vi "UltimateSerialMonitor.vi"() -> ()   [LabVIEW 2012]
uses:
  TypeDefs/StateCtrl.ctl
panel:
  in  "stop":bool
  in  "Send Command":bool
  in  "Send Serial Command":string
  out "Serial Monitor":string
  out "A5":dbl(knob) scale=0.0..10.0
  out "A4":dbl(knob) scale=0.0..10.0
  out "A3":dbl(knob) scale=0.0..10.0
  out "A2":dbl(knob) scale=0.0..10.0
  out "A1":dbl(knob) scale=0.0..10.0
  out "A0":dbl(knob) scale=0.0..10.0
  out "12":bool
  out "10":bool
  out "8":bool
  out "6":bool
  out "4":bool
  out "2":bool
  out "13":bool
  out "11":bool
  out "9":bool
  out "7":bool
  out "5":bool
  out "3":bool
  out "1":bool
  # "Analog Pins"
  # "Digital Pins"
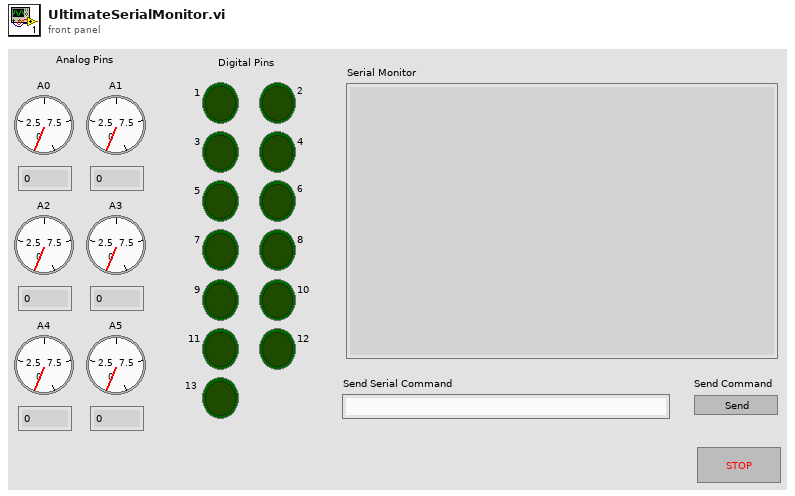
[diagram p1: front panel]
types:
  T1 = typedef "StateCtrl.ctl" = enum16{"Init", "Idle", "UpdateUI", "SendCommand", "Exit"}
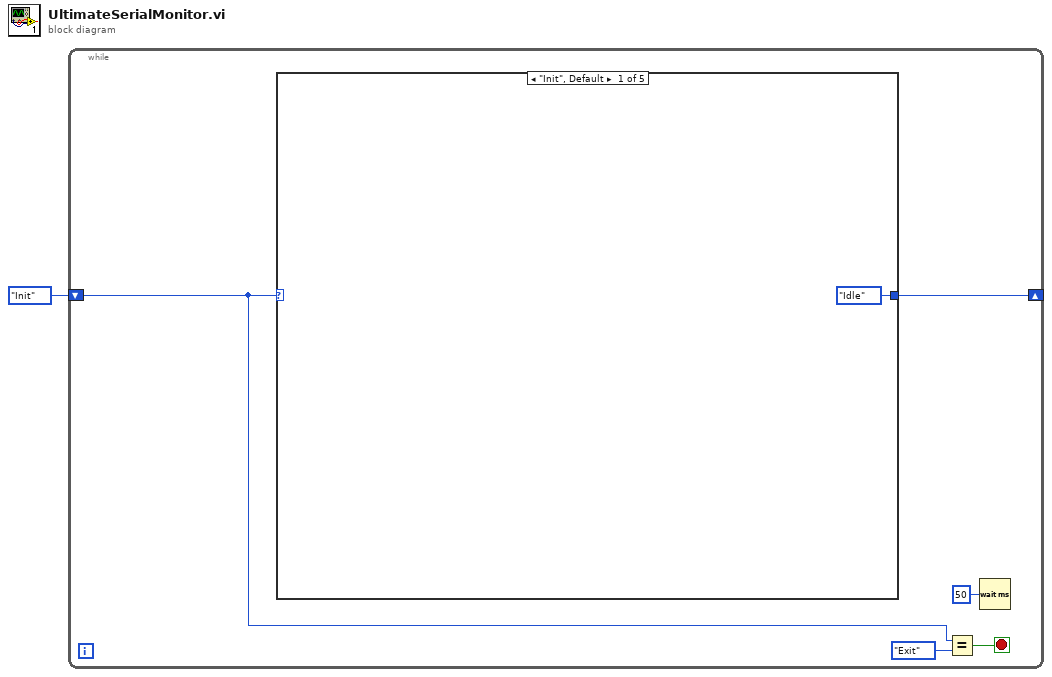
[diagram p0: block diagram]
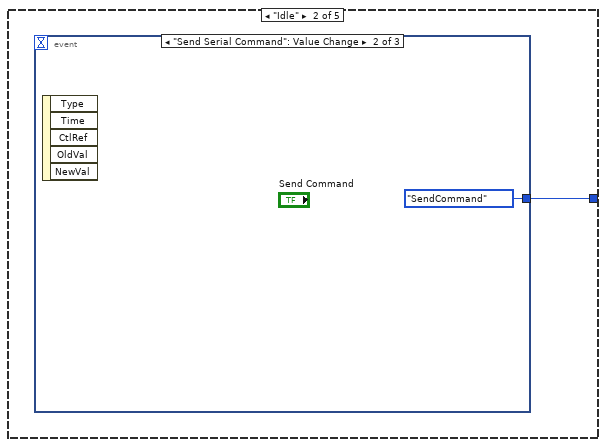
[diagram p2: hidden frame]
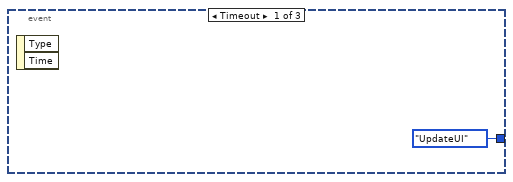
[diagram p3: hidden frame]
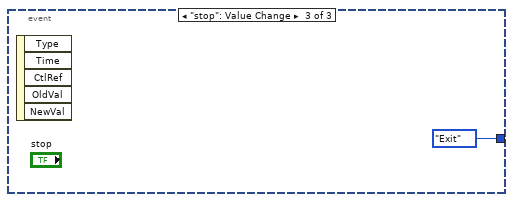
[diagram p4: hidden frame]
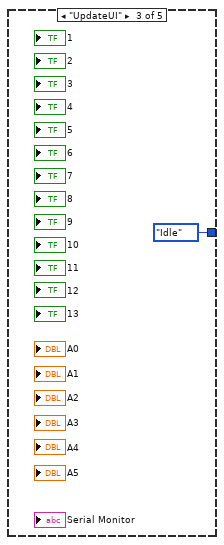
[diagram p5: hidden frame]
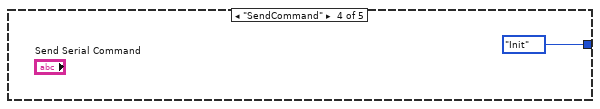
[diagram p6: hidden frame]
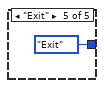
[diagram p7: hidden frame]
diagram:
  n1 = while {
    shift-right: [w6] -> _
    shift-left: StateCtrl."Init" -> [w2]
    stop <- w4 stop-if-true
    n2 = case shown="\"Init\", Default" w2 {
      tunnel: [StateCtrl."Idle" w8 StateCtrl."Idle" StateCtrl."Init" StateCtrl."Exit"] -> w6
      frame "Init", Default {
      }
      frame "Idle" {
        n3 = event shown="[1] \"Send Serial Command\": Value Change" {
          selector: _ -> [_ _ _]
          dyn-events: _ -> [_ _ _]
          timeout: _ -> [_ _ _]
          tunnel: [StateCtrl."UpdateUI" StateCtrl."SendCommand" StateCtrl."Exit"] -> w8
          event Timeout {
            n4 = event-data() -> ()  [unwired: 1 in, 2 out]
          }
          event "Send Serial Command": Value Change {
            n5 = event-data() -> ()  [unwired: 1 in, 5 out]
          }
          event "stop": Value Change {
            n6 = event-data() -> ()  [unwired: 1 in, 5 out]
          }
        }
      }
      frame "UpdateUI" {
      }
      frame "SendCommand" {
      }
      frame "Exit" {
      }
    }
    n7 = Equal?(x=w2, y=StateCtrl."Exit") -> (x = y?=w4:bool)
    n8 = Wait (ms)(milliseconds to wait=u32 50) -> ()  [unwired: 1 out]
  }
